vi "ForebrainArbiter.vi"(5 "Beh2Input":dbl[](array[numeric]), 7 "HypoInput":dbl[](array[numeric]), 11 "Beh3Input":dbl[](array[numeric])) -> (6 "ForebrainActCom":dbl[](array[numeric]))   [LabVIEW 2010]
doc: "This VI arbitrates command input from theNeo-Cortex, and Hypothallumus THINK processes and conducts a voting poll arbitor with input from each to determine the one output command.\n\nInputs: 90 cell arrays of weighted direction commands \n\nOutput: Cluster of desried velocity and direction"
uses:
  5-Forebrain/5.0-Global.vi
panel:
  out "Waveform Graph":dbl[][](graph)
  # "This subVI takes the four\nBehavior commands; three from the Neo-Cortex \nand one from theHypoThallumus and\naverages them"
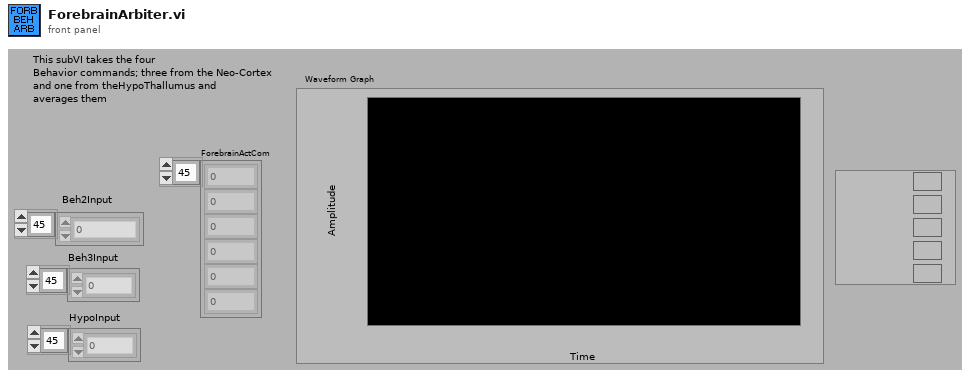
[diagram p1: front panel]
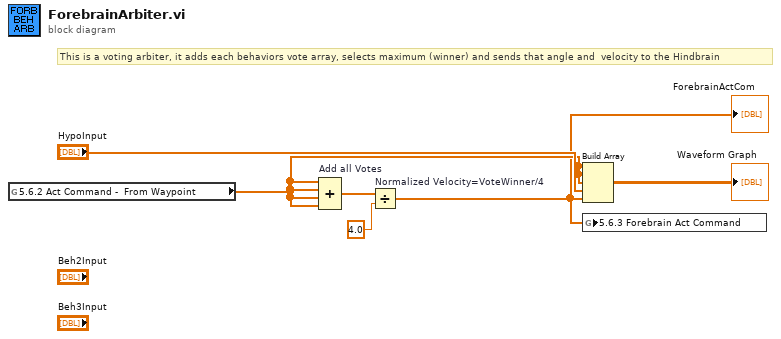
[diagram p0: block diagram]
diagram:
  # "This is a voting arbiter, it adds each behaviors vote array, selects maximum (winner) and sends that angle and  velocity to the Hindbrain"
  n1 = global read "5.0-Global.vi" "5.6.2 Act Command -  From Waypoint"() -> (w2:dbl[])
  n2 = Compound Arithmetic op=ADD "Add all Votes"(w2, w2, w2, w2) -> (w5:dbl[])
  n3 = Divide "Normalized Velocity=VoteWinner/4"(x=w5, y=4.0) -> (x/y=w1:dbl[])
  "ForebrainActCom" <- w1
  n4 = Build Array "Build Array"(w2, w2, w2, "HypoInput", w1) -> (→"Waveform Graph":dbl[][])
  n5 = global write "5.0-Global.vi" "5.6.3 Forebrain Act Command"(w1) -> ()
